vi "Add.vi"(10 "Element":T1, 11 "TypedCircularBuffer in":refnum<class "RotateCircularBuffer.lvclass">) -> (3 "TypedCircularBuffer out":refnum<class "RotateCircularBuffer.lvclass">)   [LabVIEW 2024, in "RotateCircularBuffer.lvclass"]
uses:
  RotateCircularBuffer.lvclass
  Type.ctl
  RotateCircularBuffer.lvclass/RotateCircularBuffer.ctl
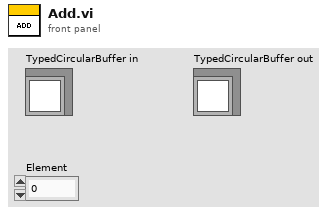
[diagram p1: front panel]
types:
  T1 = typedef "RotateCircularBuffer.lvclass/Type.ctl" = u8
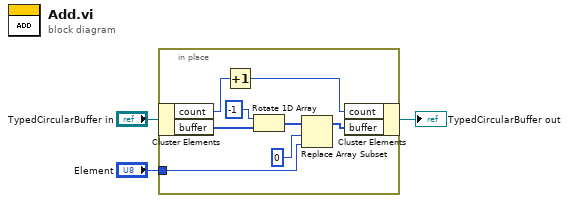
[diagram p0: block diagram]
diagram:
  n1 = in-place {
    in-place-border: "Element" -> [w10]
    n2 = in-place-cluster #1("TypedCircularBuffer in") -> ("count"=w7:u32, "buffer"=w5:T1[])
    n3 = Increment(x=w7) -> (x+1=w6:u32)
    n4 = Rotate 1D Array(1:w5, 2:-1 ("n")) -> (0:w9:T1[])
    n5 = Replace Array Subset(array=w9, new element=w10, index=0) -> (w8:T1[])
    n6 = in-place-cluster #1("count"=w6, "buffer"=w8) -> (→"TypedCircularBuffer out":refnum<class "RotateCircularBuffer.lvclass">)
  }
